vi "Mobility-Vt Calculator_Saturation_12_09_14a_PD.vi"(0 "Vg Column":dbl[](array[numeric]), 5 "Sat Id Column":dbl[](array[numeric]), 7 "NumPts":i32=5, 9 "Input Cluster":T1, 11 "Hysteresis Analysis":enum32{"1st Sweep", "2nd Sweep", "Both"}(radio)) -> (1 "Used Points":cluster{"Vg Used":dbl[], "Sqrt(Id) Used ":dbl[]}, 2 "Check Cluster":T2, 3 "Log Graph":cluster{dbl[], dbl[]}[](graph), 4 "Mobility-Sat":dbl format="%#_4e", 6 "VT-Sat":dbl, 8 "Index-Sat":i32, 10 "Sqrt Plot":cluster{dbl[], dbl[]}[](graph), 13 "Raw Graph":cluster{dbl[], dbl[]}[](graph), 14 "Off I-Sat":dbl format="%_6g", 15 "On/Off I-Sat":dbl)   [LabVIEW 2012]
uses:
  <vilib>/Analysis/NI_AALPro.lvlib
panel:
  out "Off I-Sat 2":dbl
  out "Capacitance (C)":dbl
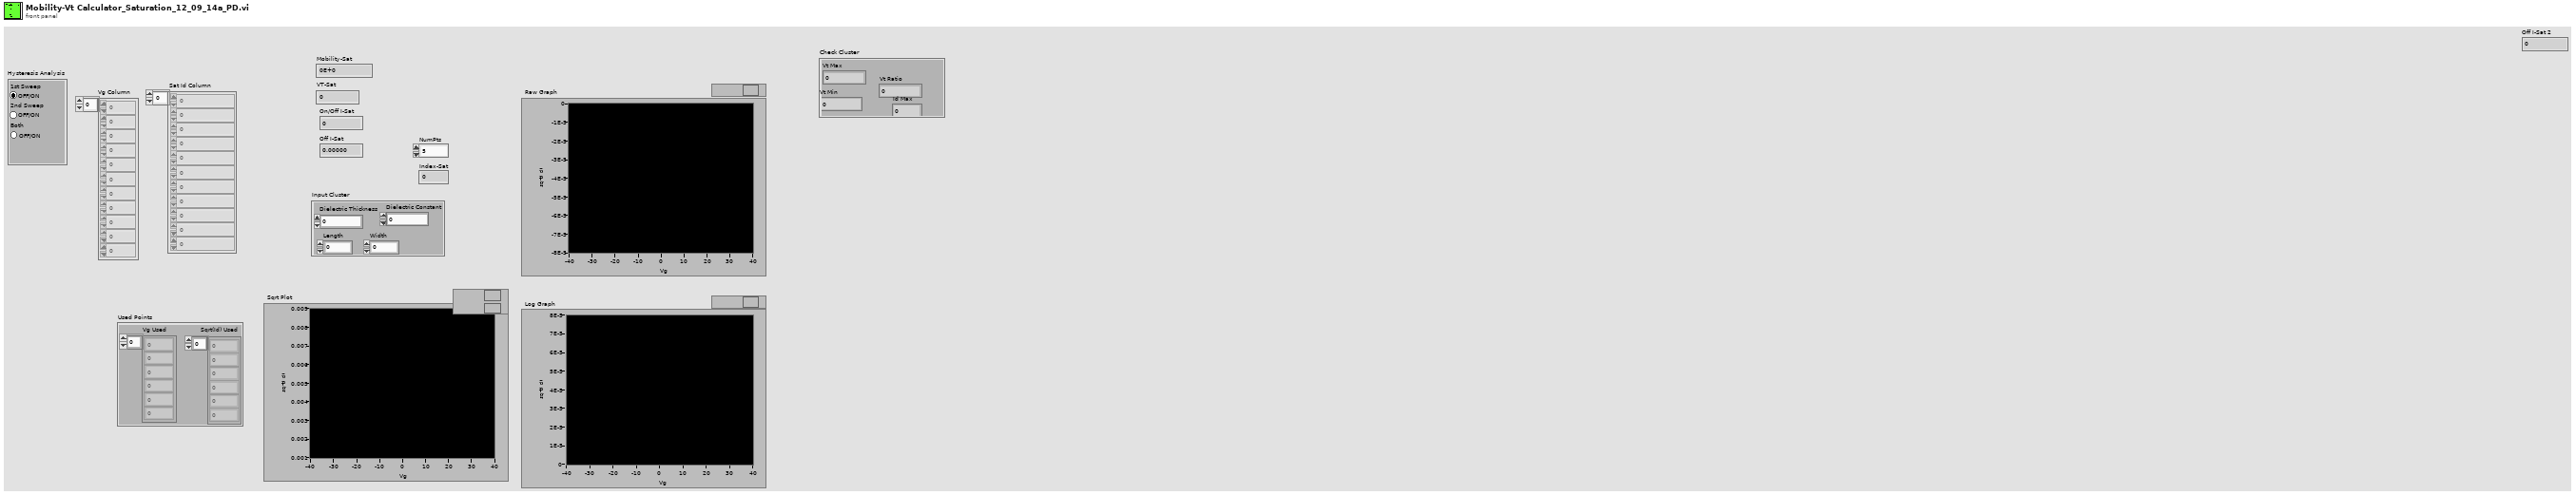
[diagram p1: front panel]
types:
  T1 = cluster{"Length":dbl, "Width":dbl, "Dielectric Thickness":dbl, "Dielectric Constant":dbl}
  T2 = cluster{"Vt Max":dbl, "Vt Min":dbl, "Vt Ratio":dbl, "Id Max":dbl}
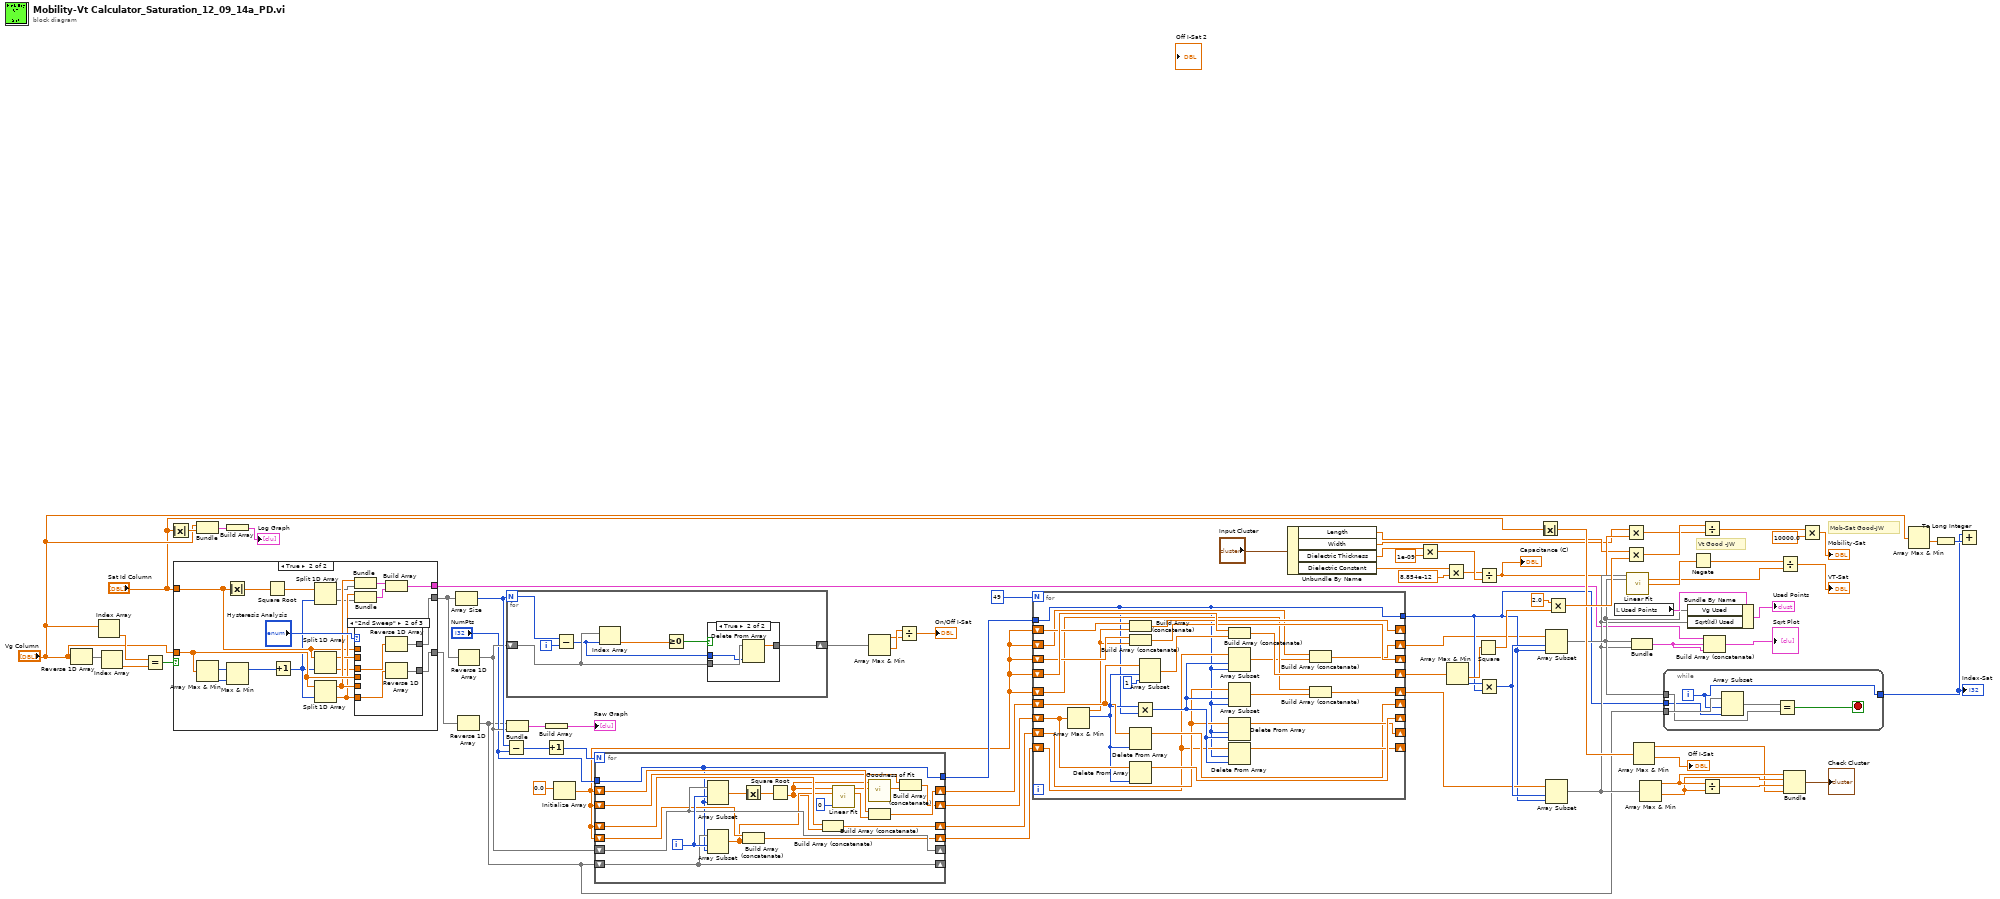
[diagram p0: block diagram]
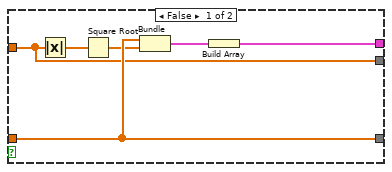
[diagram p2: hidden frame]
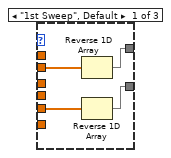
[diagram p3: hidden frame]
diagram:
  # "Mob-Sat Good-JW"
  # "Vt Good -JW"
  n1 = Reverse 1D Array(array="Vg Column") -> (reversed array=w12:dbl[])
  n2 = Index Array(array="Vg Column") -> (element=w14:dbl)  [unwired: 1 in]
  n3 = Index Array(array=w12) -> (element=w13:dbl)  [unwired: 1 in]
  n4 = Equal?(x=w14, y=w13) -> (x = y?=w11:bool)
  n5 = Absolute Value(x="Sat Id Column") -> (abs(x)=w36:dbl[])
  n6 = case shown="True" w11 {
    tunnel: "Vg Column" -> [w82 w100]
    tunnel: [w82 w99] -> w7
    tunnel: "Sat Id Column" -> [w79 w88]
    tunnel: [w79 w97] -> w8
    tunnel: [w81 w90] -> w4
    frame False {
      n7 = Absolute Value(x=w79) -> (abs(x)=w80:dbl[])
      n8 = Square Root(x=w80) -> (sqrt(x)=w78:dbl[])
      n9 = Bundle("Vg Column"=w82, w78) -> (w83:cluster{"Vg Column":dbl[], dbl[]})  [unwired: 1 in]
      n10 = Build Array(w83) -> (w81:cluster{"Vg Column":dbl[], dbl[]}[])
    }
    frame True {
      n11 = Array Max & Min(array=w100) -> (max index (indices)=w102:i32, min index (indices)=w103:i32)  [unwired: 2 out]
      n12 = Absolute Value(x=w88) -> (abs(x)=w89:dbl[])
      n13 = Max & Min(x=w102, y=w103) -> (max(x,y)=w98:i32)  [unwired: 1 out]
      n14 = Square Root(x=w89) -> (sqrt(x)=w86:dbl[])
      n15 = Increment(x=w98) -> (x+1=w87:i32)
      n16 = Split 1D Array(array=w86, index=w87) -> (first subarray=w84:dbl[], second subarray=w85:dbl[])
      n17 = Split 1D Array(array=w88, index=w87) -> (first subarray=w94:dbl[], second subarray=w92:dbl[])
      n18 = Split 1D Array(array=w100, index=w87) -> (first subarray=w95:dbl[], second subarray=w93:dbl[])
      n19 = Bundle(w95, w84) -> (w96:cluster{dbl[], dbl[]})  [unwired: 1 in]
      n20 = Bundle(w93, w85) -> (w91:cluster{dbl[], dbl[]})  [unwired: 1 in]
      n21 = case shown="\"2nd Sweep\"" "Hysteresis Analysis" {
        tunnel: w95 -> [w107 _ _]
        tunnel: w93 -> [_ w109 _]
        tunnel: w100 -> [_ _ w113]
        tunnel: [w106 w108 w113] -> w99
        tunnel: w94 -> [w105 _ _]
        tunnel: w92 -> [_ w111 _]
        tunnel: w88 -> [_ _ w112]
        tunnel: [w104 w110 w112] -> w97
        frame "1st Sweep", Default {
          n22 = Reverse 1D Array(array=w105) -> (reversed array=w104:dbl[])
          n23 = Reverse 1D Array(array=w107) -> (reversed array=w106:dbl[])
        }
        frame "2nd Sweep" {
          n24 = Reverse 1D Array(array=w111) -> (reversed array=w110:dbl[])
          n25 = Reverse 1D Array(array=w109) -> (reversed array=w108:dbl[])
        }
        frame "Both" {
        }
      }
      n26 = Build Array(w96, w91) -> (w90:cluster{dbl[], dbl[]}[])
    }
  }
  n27 = Bundle("Vg Column"="Vg Column", w36) -> (w35:cluster{"Vg Column":dbl[], dbl[]})  [unwired: 1 in]
  n28 = Build Array(w35) -> (→"Log Graph":cluster{"Vg Column":dbl[], dbl[]}[])
  n29 = Array Size(array=w8) -> (size(s)=w46:i32)
  n30 = Reverse 1D Array(array=w7) -> (reversed array=w5:dbl[])
  n31 = Reverse 1D Array(array=w8) -> (reversed array=w37:dbl[])
  n32 = Subtract(x=w46, y="NumPts") -> (x-y=w76:i32)
  n33 = for {
    N: w46 -> [w116]
    shift-right: [w119] -> w49
    shift-left: w37 -> [w120]
    i -> [w115]
    n34 = Subtract(x=w116, y=w115) -> (x-y=w114:i32)
    n35 = Index Array(array=w120, index=w114) -> (element=w117:dbl)
    n36 = Greater Or Equal To 0?(x=w117) -> (x >= 0?=w118:bool)
    n37 = case shown="True" w118 {
      tunnel: w120 -> [w121 w124]
      tunnel: w114 -> [_ w122]
      tunnel: [w121 w123] -> w119
      frame False {
      }
      frame True {
        n38 = Delete From Array(array=w124, index=w122) -> (array with subset deleted=w123:dbl[])  [unwired: 1 in, 1 out]
      }
    }
  }
  n39 = Bundle(w5, w37) -> (w39:cluster{dbl[], dbl[]})  [unwired: 1 in]
  n40 = Increment(x=w76) -> (x+1=w77:i32)
  n41 = Build Array(w39) -> (→"Raw Graph":cluster{dbl[], dbl[]}[])
  n42 = Initialize Array(0.0) -> (w3:dbl[])  [unwired: 1 in]
  n43 = for {
    N: w77 -> [_]
    shift-right: [w130] -> _
    shift-left: w5 -> [w130]
    shift-right: [w138] -> _
    shift-left: w37 -> [w138]
    shift-right: [w142] -> w66
    shift-left: w3 -> [w141]
    shift-right: [w140] -> w68
    shift-left: w3 -> [w139]
    tunnel: "NumPts" -> [w125]
    shift-right: [w133] -> w71
    shift-left: w3 -> [w134]
    shift-right: [w131] -> w72
    shift-left: w3 -> [w132]
    tunnel: [w125] -> w21
    i -> [w144]
    n44 = Array Subset(array=w138, index=w144, length=w125) -> (w137:dbl[])
    n45 = Array Subset(array=w130, index=w144, length=w125) -> (w129:dbl[])
    n46 = Absolute Value(x=w137) -> (abs(x)=w136:dbl[])
    n47 = Build Array (concatenate)(w132, w129) -> (w131:dbl[])
    n48 = Square Root(x=w136) -> (sqrt(x)=w126:dbl[])
    n49 = Build Array (concatenate)(w134, w126) -> (w133:dbl[])
    n50 = call <vilib>:"Linear Fit.vi"("Y"=w126, "X"=w129, "method"=0) -> ("Best Linear Fit"=w128:dbl[], "slope"=w143:dbl)  [unwired: 8 in, 3 out]
    n51 = call <vilib>:"Goodness of Fit.vi"("Best Fit"=w128, "Y"=w126) -> ("R-square"=w127:dbl)  [unwired: 6 in, 3 out]
    n52 = Build Array (concatenate)(w141, w143) -> (w142:dbl[])
    n53 = Build Array (concatenate)(w139, w127) -> (w140:dbl[])
  }
  n54 = Array Max & Min(array=w49) -> (max value=w47:dbl, min value=w48:dbl)  [unwired: 2 out]
  n55 = Divide(x=w48, y=w47) -> (x/y=→"On/Off I-Sat":dbl)
  n56 = for {
    N: 49 -> [_]
    shift-right: [w169] -> _
    shift-left: w68 -> [w170]
    shift-right: [w150] -> _
    shift-left: w66 -> [w151]
    shift-right: [w166] -> w67
    shift-left: w3 -> [w165]
    shift-right: [w164] -> _
    shift-left: w3 -> [w163]
    shift-right: [w162] -> _
    shift-left: w3 -> [w161]
    shift-right: [w160] -> _
    shift-left: w71 -> [w147]
    shift-right: [w158] -> _
    shift-left: w72 -> [w146]
    tunnel: w21 -> [w145]
    shift-right: [w157] -> w73
    shift-left: w3 -> [w156]
    shift-right: [w155] -> w2
    shift-left: w3 -> [w154]
    tunnel: [w145] -> w20
    n57 = Array Max & Min(array=w170) -> (max value=w149:dbl, max index (indices)=w148:i32)  [unwired: 2 out]
    n58 = Build Array (concatenate)(w161, w149) -> (w162:dbl[])
    n59 = Build Array (concatenate)(w163, w149) -> (w164:dbl[])
    n60 = Delete From Array(array=w151, index=w148) -> (array with subset deleted=w150:dbl[])  [unwired: 1 in, 1 out]
    n61 = Delete From Array(array=w170, index=w148) -> (array with subset deleted=w169:dbl[])  [unwired: 1 in, 1 out]
    n62 = Multiply(x=w148, y=w145) -> (x*y=w159:i32)
    n63 = Array Subset(array=w151, index=w148, length=1) -> (w167:dbl[])
    n64 = Build Array (concatenate)(w165, w167) -> (w166:dbl[])
    n65 = Array Subset(array=w146, index=w159, length=w145) -> (w153:dbl[])
    n66 = Array Subset(array=w147, index=w159, length=w145) -> (w152:dbl[])
    n67 = Delete From Array(array=w147, length=w145, index=w159) -> (array with subset deleted=w160:dbl[])  [unwired: 1 out]
    n68 = Delete From Array(array=w146, length=w145, index=w159) -> (array with subset deleted=w158:dbl[])  [unwired: 1 out]
    n69 = Build Array (concatenate)(w154, w153) -> (w155:dbl[])
    n70 = Build Array (concatenate)(w156, w152) -> (w157:dbl[])
  }
  n71 = Unbundle By Name("Input Cluster") -> ("Length"=w16:dbl, "Width"=w15:dbl, "Dielectric Thickness"=w17:dbl, "Dielectric Constant"=w18:dbl)
  n72 = Multiply(x=w17, y=1e-09) -> (x*y=w52:dbl)
  n73 = Multiply(x=w18, y=8.854e-12) -> (x*y=w50:dbl)
  n74 = Array Max & Min(array=w67) -> (min value=w64:dbl, min index (indices)=w74:i32)  [unwired: 2 out]
  n75 = Square(x=w64) -> (x^2=w63:dbl)
  n76 = Divide(x=w50, y=w52) -> (x/y=w27:dbl)
  "Capacitance (C)" <- w27
  n77 = Multiply(x=w74, y=w20) -> (x*y=w75:i32)
  n78 = Absolute Value(x="Sat Id Column") -> (abs(x)=w45:dbl[])
  n79 = Array Subset(array=w2, index=w75, length=w20) -> (w31:dbl[])
  n80 = Array Subset(array=w73, index=w75, length=w20) -> (w30:dbl[])
  n81 = Multiply(x=2.0, y=w63) -> (x*y=w62:dbl)
  n82 = local read "Used Points"() -> (w33:cluster{"Vg Used":dbl[], "Sqrt(Id) Used ":dbl[]})
  n83 = Multiply(x=w15, y=w27) -> (x*y=w60:dbl)
  n84 = Multiply(x=w16, y=w62) -> (x*y=w61:dbl)
  n85 = call <vilib>:"Linear Fit.vi"("Y"=w30, "X"=w31) -> ("slope"=w54:dbl, "intercept"=w56:dbl)  [unwired: 9 in, 3 out]
  n86 = Bundle(w31, w30) -> (w1:cluster{dbl[], dbl[]})  [unwired: 1 in]
  n87 = Array Max & Min(array=w45) -> (max value=w40:dbl, min value=→"Off I-Sat":dbl)  [unwired: 2 out]
  n88 = Array Max & Min(array=w30) -> (max value=w44:dbl, min value=w43:dbl)  [unwired: 2 out]
  n89 = while {
    tunnel: w5 -> [w175]
    tunnel: w31 -> [w172]
    tunnel: [w173] -> w6
    tunnel: w20 -> [w171]
    i -> [w173]
    stop <- w176 stop-if-true
    n90 = Array Subset(array=w175, index=w173, length=w171) -> (w174:dbl[])
    n91 = Equal?(x=w174, y=w172) -> (x = y?=w176:bool)
  }
  "Index-Sat" <- w6
  n92 = Bundle By Name(cluster=w33, "Vg Used"=w31, "Sqrt(Id) Used"=w30) -> (→"Used Points":cluster{"Vg Used":dbl[], "Sqrt(Id) Used ":dbl[]})
  n93 = Negate(x=w56) -> (-x=w55:dbl)
  n94 = Divide(x=w61, y=w60) -> (x/y=w58:dbl)
  n95 = Divide(x=w44, y=w43) -> (x/y=w42:dbl)
  n96 = Build Array (concatenate)(w4, w1, w1) -> (→"Sqrt Plot":cluster{"Vg Column":dbl[], dbl[]}[])
  n97 = Divide(x=w55, y=w54) -> (x/y=→"VT-Sat":dbl)
  n98 = Bundle(w44, w43, w42, w40) -> (→"Check Cluster":cluster{dbl, dbl, dbl, dbl})  [unwired: 1 in]
  n99 = Multiply(x=w58, y=10000.0) -> (x*y=→"Mobility-Sat":dbl)
  n100 = Array Max & Min(array="Vg Column") -> (min value=w29:dbl)  [unwired: 3 out]
  n101 = To Long Integer(number=w29) -> (32bit integer=w28:i32)
  n102 = Add(x=w6, y=w28) -> ()  [unwired: 1 out]
